vi "Store to Memory.vi"(8 "error in (no error)":errorcluster, 9 "Destination (0: Memory 1)":u16(ring) items=["Memory 1", "Memory 2", "Memory 3", "Memory 4", "File"], 10 "Source (0: Channel 1)":u16(ring) items=["Channel 1", "Channel 2", "Channel 3", "Channel 4", "Memory 1", "Memory 2", "Memory 3", "Memory 4", "Function 1", "Function 2", "Function 3", "Function 4", "Function 5", "Function 6", "Function 7", "Function 8"], 11 "VISA resource name":refnum<visa-resource-name>) -> (0 "error out":errorcluster, 3 "VISA resource name out":refnum<visa-resource-name>)   [LabVIEW 2015, in "LeCroy Wave Series.lvlib"]
doc: "Store the waveform the oscilloscope acquired for the specified channel to the specified destination.\n\nNote:\nThis VI has been obsoleted from the driver and is included for compatibility with existing applications. New applications should use the Save Waveform VI."
uses:
  <instrlib>/LeCroy Wave Series/LeCroy Wave Series.lvlib
panel:
  # "Note:\nThis VI has been obsoleted from the driver and is included for compatibility with existing applications.  New applications should use the Save Waveform VI."
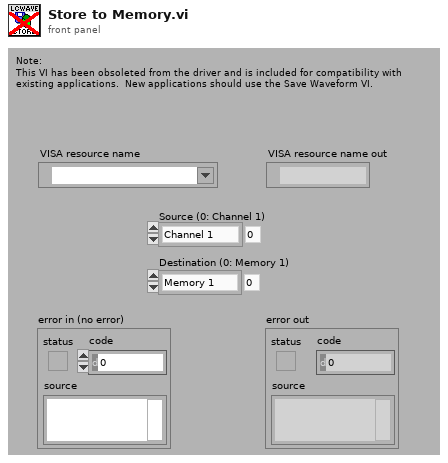
[diagram p1: front panel]
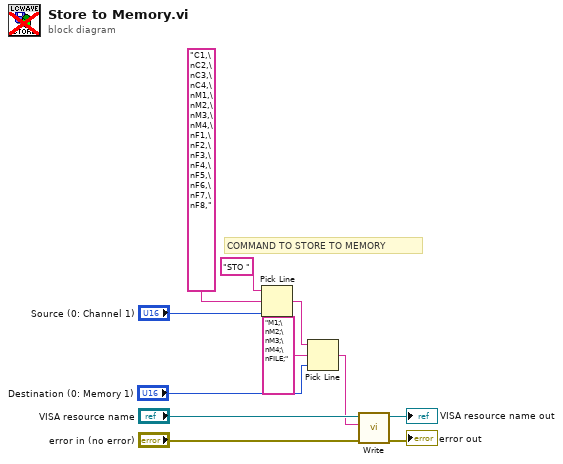
[diagram p0: block diagram]
diagram:
  # "COMMAND TO STORE TO MEMORY"
  n1 = Pick Line(string ("")="STO ", multi-line string="C1,\nC2,\nC3,\nC4,\nM1,\nM2,\nM3,\nM4,\nF1,\nF2,\nF3,\nF4,\nF5,\nF6,\nF7,\nF8,", line index="Source (0: Channel 1)") -> (output string=w3:string)
  n2 = Pick Line(string ("")=w3, multi-line string="M1;\nM2;\nM3;\nM4;\nFILE;", line index="Destination (0: Memory 1)") -> (output string=w2:string)
  n3 = call <instrlib>:"Write.vi"("error in (no error)"="error in (no error)", "Write Buffer"=w2, "VISA resource name"="VISA resource name") -> ("error out"=→"error out":errorcluster, "VISA resource name out"=→"VISA resource name out":refnum<visa-resource-name>)  [unwired: 6 in, 1 out]
